vi "VerifyArgumentsCore.vi"(8 "error in (no error)":errorcluster, 11 "ExecuteBuildSpecAllTargets in":refnum<class "ExecuteBuildSpecAllTargets.lvclass">) -> (0 "error out":errorcluster, 3 "ExecuteBuildSpecAllTargets out":refnum<class "ExecuteBuildSpecAllTargets.lvclass">)   [LabVIEW 2020, in "ExecuteBuildSpecAllTargets.lvclass"]
doc: "Ensures required arguments are provided to the LabVIEWCLI."
uses:
  ExecuteBuildSpecAllTargets.lvclass
  Program Files (x86)/National Instruments/Shared/LabVIEW CLI/Operations/Utilities/OperationErrorType.ctl
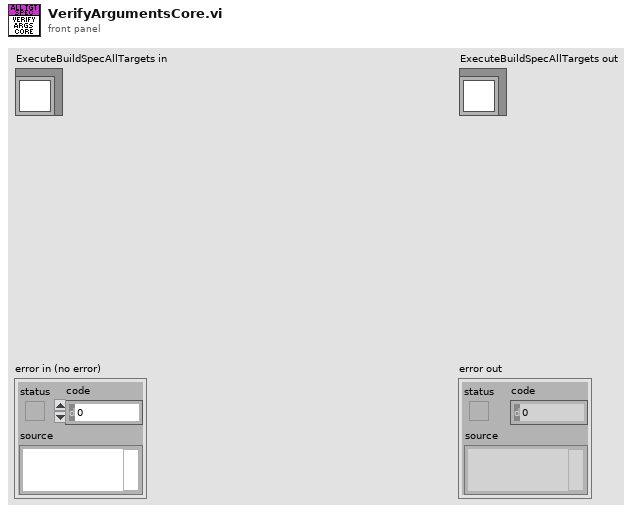
[diagram p1: front panel]
types:
  T1 = typedef "OperationErrorType.ctl" = enum16{"RequiredArgumentMissing", "UnknownArguments", "LoggerSetMultipleTimes", "OperationBrokenError"}
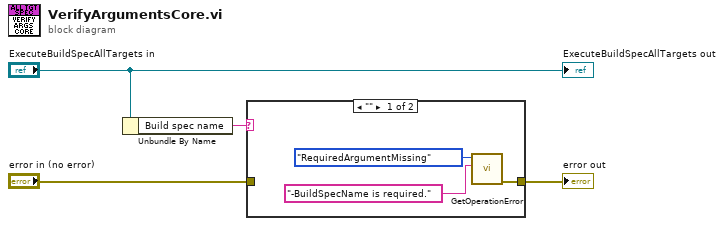
[diagram p0: block diagram]
diagram:
  n1 = Unbundle By Name("ExecuteBuildSpecAllTargets in") -> ("Build spec name"=w4:string)
  n2 = case shown="\"\"" w4 {
    tunnel: [w7 w8] -> w3
    tunnel: "error in (no error)" -> [_ w8]
    frame "" {
      n3 = call "GetOperationError.vi"("Additional Information"="-BuildSpecName is required.", "Operation Error Type"=OperationErrorType."RequiredArgumentMissing") -> ("error out"=w7:errorcluster)  [unwired: 9 in]
    }
    frame Default {
    }
  }
  "error out" <- w3
  "ExecuteBuildSpecAllTargets out" <- "ExecuteBuildSpecAllTargets in"
